vi "RTC闹钟实验.vi"   [LabVIEW 2011]
uses:
  <vilib>/STM32_DriverVI_Interface_F4/Timer/TIMX Interrupt_F4.ctl
  <vilib>/STM32_DriverVI_Interface_F4/Interrupt/PreemptionPriority_2_F4.ctl
  <vilib>/STM32_DriverVI_Interface_F4/Interrupt/SubPriority_2_F4.ctl
  <vilib>/STM32_DriverVI_Interface_F4/RTC/RTC_ClK_Source_F4xx.ctl
  <vilib>/STM32_DriverVI_Interface_F4/RTC/RTC_Set_Alarm_A_Week_F4.vi
  <vilib>/STM32_DriverVI_Interface_F4/Timer/TIM Priority Set_2_F4.vi
types:
  T1 = typedef "允许或禁止PWM输出_F4.ctl" = enum8{"禁止", "允许"}
  T2 = typedef "RTC中断类型_F4.ctl" = enum8{"Alarm A Interrupt", "Alarm B Interrupt", "RTC WKUP（Overflow） Int"}
  T3 = typedef "SubPriority_2_F4.ctl" = enum8{"Priority_0（High）", "Priority_1", "Priority_2", "Priority_3（Low）"}
  T4 = typedef "PreemptionPriority_2_F4.ctl" = enum8{"Priority_0（Highest）", "Priority_1", "Priority_2", "Priority_3（Lowest）"}
  T5 = typedef "TIMX Interrupt_F4.ctl" = u8
  T6 = typedef "中断使能禁止_F4.ctl" = enum8{"Disable", "Enable"}
  T7 = typedef "RTC计数时钟频率_F4.ctl" = u8
  T8 = typedef "RTC_ClK_Source_F4xx.ctl" = enum8{"外部:32.768KHz", "内部:LSI: 40KHz"}
  T9 = enum8{"None", "Monday", "Tuesday", "Wednesday", "Thursday", "Friday", "Saturday", "Sunday"}
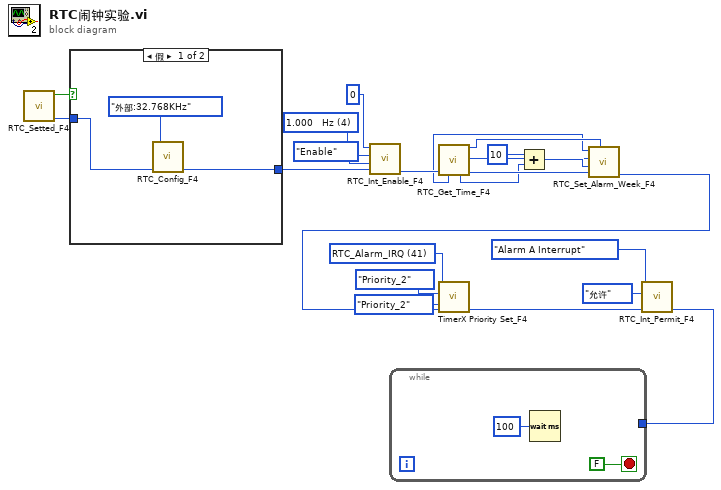
[diagram p0: block diagram]
diagram:
  w8 = T5 41 items=["WWDG_IRQ"=0, "RTC_WKUP_IRQ"=3, "RTC_Alarm_IRQ"=41, "TIM1_BRK_TIM9_IRQ"=24, "TIM1_UP_TIM10_IRQ"=25, "TIM1_TRG_COM_TIM11_IRQ"=26, "TIM1_CC_IRQ"=27, "TIM2_IRQ"=28, "TIM3_IRQ"=29, "TIM4_IRQ"=30, "TIM5_IRQ"=50, "TIM6_IRQ"=54, "TIM7_IRQ"=55, "TIM8_BRK_TIM12_IRQ"=43, "TIM8_UP_TIM13_IRQ"=44, "TIM8_TRG_COM_TIM14_IRQ"=45, "TIM8_CC_IRQ"=46] ("TIM 中断号设置")
  w18 = T7 4 items=["16.384 KHz"=3, "8.192   KHz"=2, "4.096   KHz"=1, "2.048   KHz"=0, "1.000   Hz"=4] ("时钟预分频数")
  n1 = call <vilib>:"RTC_Setted_F4.vi"() -> ("err_out"=w21:u8, "RTC是否已经设置过？"=w22:bool)  [unwired: 10 in]
  n2 = case shown="假" w22 {
    tunnel: w21 -> [w25 _]
    tunnel: [w23 _] -> w20
    frame False {
      n3 = call <vilib>:"RTC_Config_F4.vi"("err_in"=w25, "RTC_CLK_Source_F4"=RTC_ClK_Source_F4xx."外部:32.768KHz") -> ("err_out"=w23:u8)  [unwired: 8 in, 1 out]
    }
    frame True {
    }
  }
  n4 = call <vilib>:"RTC_Int_Enable_F4.vi"("err_in"=w20, "RTC时钟开启/关闭"=中断使能禁止_F4."Enable", "时钟预分频数"=w18, "自动重装值"=u16 0) -> ("err_out"=w16:u8)  [unwired: 7 in]
  n5 = call <vilib>:"RTC_Get_Time_F4.vi"("err_in"=w16) -> ("Week"=w11:T9, "Hour"=w10:u8, "Minute"=w9:u8, "Second"=w13:u8, "err_out"=w15:u8)  [unwired: 6 in, 4 out]
  n6 = Add(x=u8 10, y=w13) -> (x+y=w14:u8)
  n7 = call-poly <vilib>:"RTC_Set_Alarm_Week_F4.vi"("Week"=w11, "err_in"=w15, "Second"=w14, "Minute"=w9, "Hour"=w10) -> ("err_out"=w5:u8)  [unwired: 6 in]
  n8 = call-poly <vilib>:"TimerX Priority Set_F4.vi"("err_in"=w5, "响应优先级"=SubPriority_2_F4."Priority_2", "抢占优先级"=PreemptionPriority_2_F4."Priority_2", "IO 中断号设置"=w8) -> ("err_out"=w4:u8)  [unwired: 6 in, 1 out]
  n9 = call <vilib>:"RTC_Int_Permit_F4.vi"("err_in"=w4, "RTC中断允许"=允许或禁止PWM输出_F4."允许", "RTC中断类型"=RTC中断类型_F4."Alarm A Interrupt") -> ("err_out"=w1:u8)  [unwired: 8 in]
  n10 = while {
    tunnel: w1 -> [_]
    stop <- FALSE stop-if-true
    n11 = Wait (ms)(milliseconds to wait=u32 100 ("等待时间（毫秒）")) -> ()  [unwired: 1 out]
  }
